vi "UnbundleName_NoName.vi"() -> ()   [LabVIEW 2021]
panel:
  out "Release Date 2":dbl
  out "Director 2":string
  out "Movie Title 2":string
  out "Release Date":dbl
  out "Director":string
  out "Movie Title":string
  in  "Cluster":T1
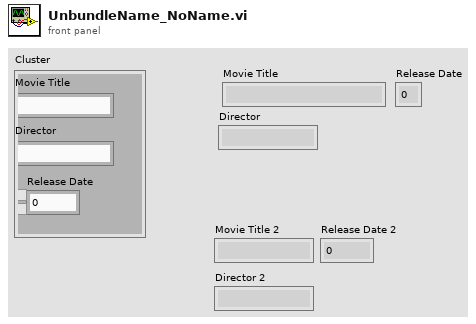
[diagram p1: front panel]
types:
  T1 = cluster{"Movie Title":string, "Director":string, "Release Date":dbl}
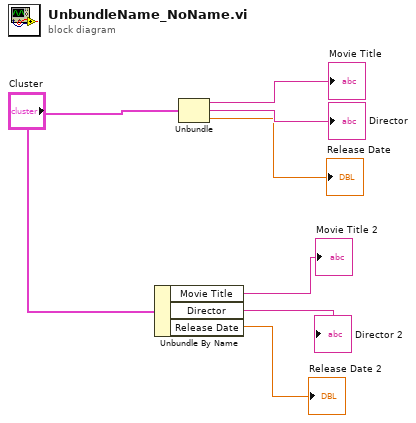
[diagram p0: block diagram]
diagram:
  n1 = Unbundle By Name("Cluster") -> ("Movie Title"=→"Movie Title 2":string, "Director"=→"Director 2":string, "Release Date"=→"Release Date 2":dbl)
  n2 = Unbundle("Cluster") -> ("Movie Title"=→"Movie Title":string, "Director"=→"Director":string, "Release Date"=→"Release Date":dbl)
